vi "XY Graph Show-Hide Grid Event.vi"(8 "Error In":errorcluster, 11 "XYGraph Ref in":T1) -> (0 "Error Out":errorcluster, 1 "Message":string, 2 "Grid Shown?":bool, 3 "XYGraph Ref out":T1)   [LabVIEW 2019, in "XY Graph Add-Ons.lvlib"]
uses:
  XY Graph Add-Ons.lvlib
  XY Graph Refnum.ctl
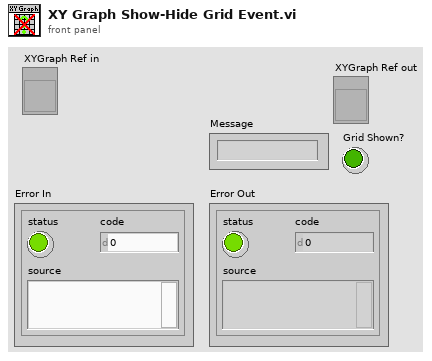
[diagram p1: front panel]
types:
  T1 = typedef "XY Graph Add-Ons.lvlib/XY Graph Refnum.ctl" = refnum<vi>
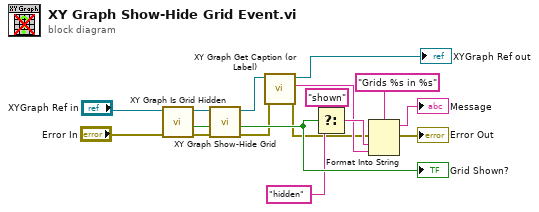
[diagram p0: block diagram]
diagram:
  n1 = call "XY Graph Is Grid Hidden.vi"("Error In"="Error In", "XY Graph Ref"="XYGraph Ref in") -> ("Error Out (dup)"=w16:errorcluster, "Hidden Grid(s)"=w17:bool, "XY Graph Ref out"=w5:T1)  [unwired: 7 in]
  n2 = call "XY Graph Show-Hide Grid.vi"("Error In"=w16, "Hide (F) /Show (T)"=w17, "XYGraph Ref"=w5) -> ("Error Out"=w3:errorcluster, "Grid Shown?"=w11:bool, "XYGraph Ref out"=w4:T1)  [unwired: 6 in]
  "Grid Shown?" <- w11
  n3 = call "XY Graph Get Caption (or Label).vi"("error in (no error)"=w3, "XYGraph in"=w4) -> ("error out"=w2:errorcluster, "Caption (or Label) Text"=w6:string, "XYGraph out"=→"XYGraph Ref out":T1)  [unwired: 7 in]
  n4 = Select(t="shown" ("format string"), s=w11, f="hidden" ("format string")) -> (s? t:f=w8:string)
  n5 = Format Into String(format string="Grids %s in %s", error in=w2, w8, w6) -> (resulting string=→"Message":string, error out=→"Error Out":errorcluster)  [unwired: 1 in]
